vi "Read LINX I2C Channel.vi"(8 "error in (no error)":errorcluster, 11 "LINX-PCA9865 PWM in":refnum<class "LINX-PCA9865 PWM.lvclass">) -> (0 "error out":errorcluster, 2 "LINX I2C Channel":u8=1, 3 "LINX-PCA9865 PWM out":refnum<class "LINX-PCA9865 PWM.lvclass">)   [LabVIEW 2019, in "LINX-PCA9865 PWM.lvclass"]
uses:
  LINX-PCA9865 PWM.lvclass
  LINX-PCA9865 PWM.lvclass/LINX-PCA9865 PWM.ctl
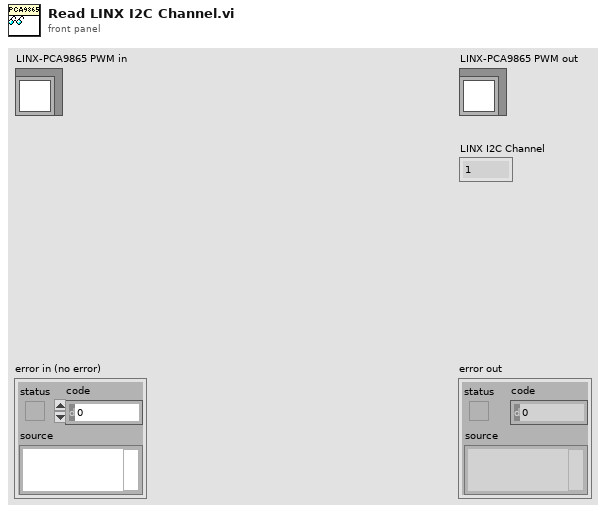
[diagram p1: front panel]
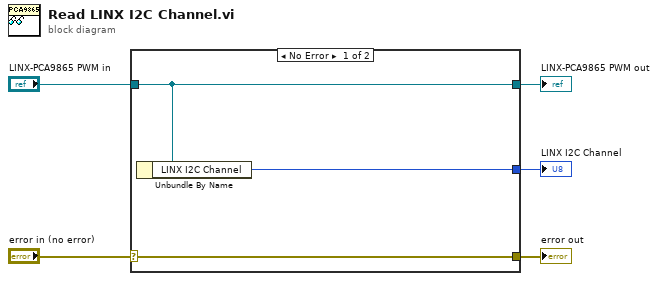
[diagram p0: block diagram]
diagram:
  n1 = case shown="No Error" "error in (no error)" {
    selector: "error in (no error)" -> [w8 w9]
    tunnel: [w8 w9] -> w4
    tunnel: [w7 w10] -> w2
    tunnel: "LINX-PCA9865 PWM in" -> [w7 w10]
    tunnel: [w6 _] -> w1
    frame No Error {
      n2 = Unbundle By Name(w7) -> ("LINX I2C Channel"=w6:u8)
    }
    frame Error {
    }
  }
  "error out" <- w4
  "LINX-PCA9865 PWM out" <- w2
  "LINX I2C Channel" <- w1
